vi "Convert Cluster to Waveforms.vi"(0 "data block":T1, 1 "physical channels":T2[](array[typedef])=[enum."Voltage Phase A (L1)", enum."Voltage Phase B (L2)", enum."Voltage Phase C (L3)", enum."Current Phase A (L1)", enum."Current Phase B (L2)", enum."Current Phase C (L3)", enum."Current Phase N (Neutral)"], 2 "reset? (F)":bool, 9 "system info in":refnum<class "EP System Info.lvclass">, 11 "error in (no error)":errorcluster) -> (4 "voltage waveforms":waveform(dbl)[](array[waveform]), 6 "current waveforms":waveform(dbl)[](array[waveform]), 10 "system info out":refnum<class "EP System Info.lvclass">, 14 "interval length [s]":dbl, 15 "error out":errorcluster)   [LabVIEW 2014, in "NI_EP_Power Quality.lvlib"]
doc: "Converts resampled voltage and current data to voltage and current waveforms of different line configurations. This VI also arranges the order of the elements in the waveforms of each three-phase electrical power system for further measurement. For example, the orders are A-B-C-N for the four-channel method and A-B-C for the three-channel method. You must manually select the polymorphic instance you want to use."
uses:
  <vilib>/addons/Electrical Power/PQ/NI_EP_Power Quality.lvlib
  <vilib>/addons/Electrical Power/PQ/Common/Classes/System Info/EP System Info.lvclass
  <vilib>/addons/Electrical Power/PQ/Common/Controls/ep_AI Data Channel.ctl
  <vilib>/addons/Electrical Power/PQ/Resampling/Desktop/subVIs/ep_Resampled Data.ctl
  <vilib>/addons/Electrical Power/PQ/Resampling/NI_EP_Resample_Host.lvlib
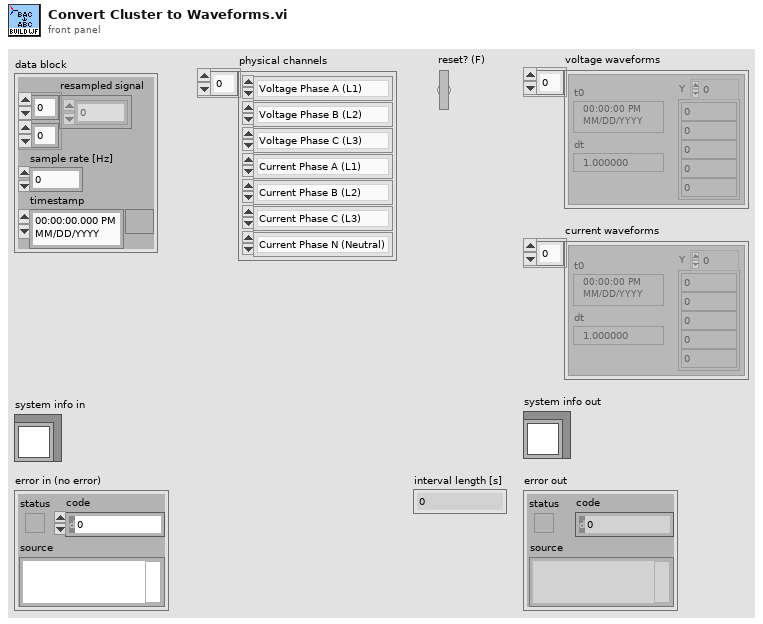
[diagram p1: front panel]
types:
  T1 = typedef "NI_EP_Resample_Host.lvlib/ep_Resampled Data.ctl" = cluster{"resampled signal":dbl[][], "sample rate [Hz]":dbl, "timestamp":timestamp}
  T2 = typedef "NI_EP_Power Quality.lvlib/ep_AI Data Channel.ctl" = enum16{"Voltage Phase A (L1)", "Voltage Phase B (L2)", "Voltage Phase C (L3)", "Voltage Phase N (Neutral)", "Current Phase A (L1)", "Current Phase B (L2)", "Current Phase C (L3)", "Current Phase N (Neutral)"}
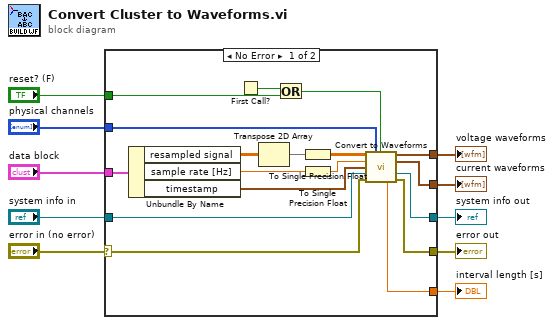
[diagram p0: block diagram]
diagram:
  n1 = case shown="No Error" "error in (no error)" {
    selector: "error in (no error)" -> [w18 w30]
    tunnel: "physical channels" -> [w22 _]
    tunnel: [w17 w30] -> w9
    tunnel: [w16 w29] -> w8
    tunnel: "reset? (F)" -> [w27 _]
    tunnel: "system info in" -> [w19 w29]
    tunnel: "data block" -> [w26 _]
    tunnel: [w21 _] -> w3
    tunnel: [w20 _] -> w2
    tunnel: [w15 _] -> w1
    frame No Error {
      n2 = Unbundle By Name(w26) -> ("resampled signal"=w24:dbl[][], "sample rate [Hz]"=w12:dbl, "timestamp"=w23:timestamp)
      n3 = First Call?() -> (First Call?: T/F=w28:bool)
      n4 = Transpose 2D Array(2D array=w24) -> (transposed array=w13:dbl[][])
      n5 = Or(x=w28, y=w27) -> (x .or. y?=w25:bool)
      n6 = To Single Precision Float(number=w13) -> (single precision float=w14:sgl[][])
      n7 = To Single Precision Float(number=w12) -> (single precision float=w11:sgl)
      n8 = call <vilib>:"Convert to Waveforms.vi"("data in"=w14, "physical channels"=w22, "reset? (F)"=w25, "sample rate [Hz]"=w11, "timestamp"=w23, "system info in"=w19, "error in (no error)"=w18) -> ("voltage waveforms"=w21:waveform(dbl)[], "current waveforms"=w20:waveform(dbl)[], "system info out"=w16:refnum<class "EP System Info.lvclass">, "interval length [s]"=w15:dbl, "error out"=w17:errorcluster)  [unwired: 4 in]
    }
    frame Error {
    }
  }
  "voltage waveforms" <- w3
  "error out" <- w9
  "current waveforms" <- w2
  "system info out" <- w8
  "interval length [s]" <- w1
